vi "test_generic.vi"() -> ()   [LabVIEW 2010, in "GenericClock.lvclass"]
uses:
  GenericClock.lvclass
  common/classes/GenericComponent/GenericComponent/GenericComponent.lvclass
panel:
  in  "duty cycle":dbl[unit]
  in  "duration high":dbl[unit]
  in  "offset":dbl[unit]
  in  "create button":bool
  out "error out":errorcluster
  in  "stop":bool
  in  "start":bool
  in  "number of repetitions":i64=1000000000
  in  "pulse frequency":dbl[unit]=80000.0
  # "Test GenericClock"
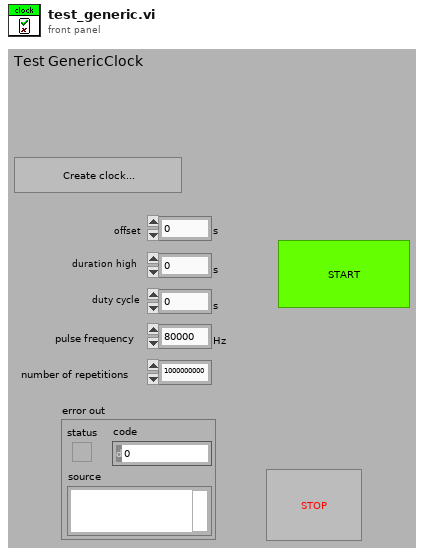
[diagram p1: front panel]
types:
  T1 = typedef "XComponentSpecification.xctl/data.ctl" = cluster{"class path":string, "configuration":string, "label":string, "settings name":string}
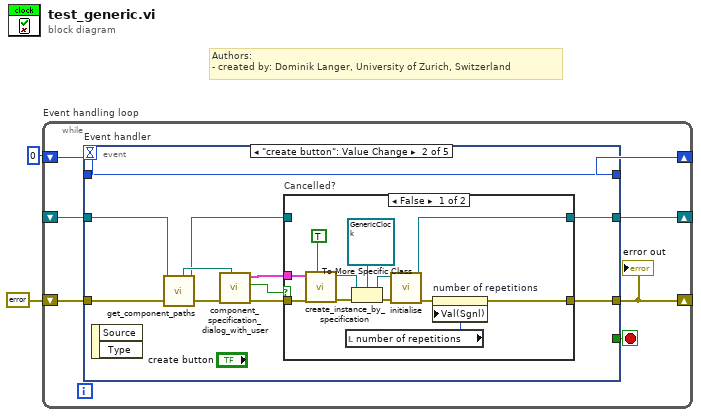
[diagram p0: block diagram]
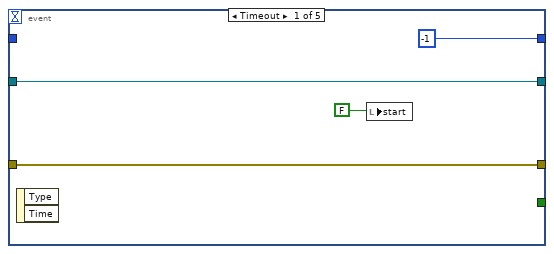
[diagram p2: hidden frame]
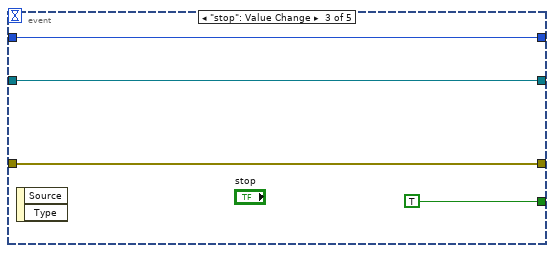
[diagram p4: hidden frame]
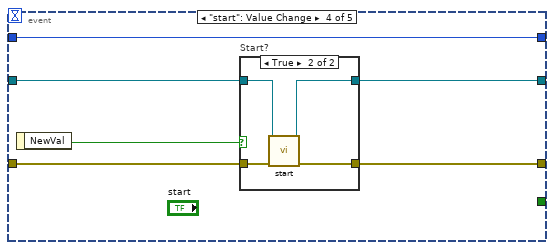
[diagram p5: hidden frame]
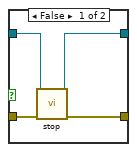
[diagram p6: hidden frame]
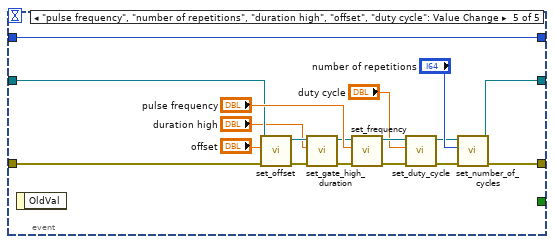
[diagram p7: hidden frame]
diagram:
  # "Authors: \n- created by: Dominik Langer, University of Zurich, Switzerland"
  n1 = while "Event handling loop" {
    shift-right: [w6] -> _
    shift-left: errorcluster {"status"=FALSE, "code"=0, "source"=""} ("error out") -> [w7]
    shift-right: [w5] -> _
    shift-left: _ -> [w9]
    shift-right: [w4] -> _
    shift-left: 0 -> [w8]
    stop <- w3 stop-if-true
    n2 = event "Event handler" shown="[1] \"create button\": Value Change" {
      selector: _ -> [_ _ _ _ _]
      dyn-events: _ -> [_ _ _ _ _]
      timeout: w8 -> [_ _ _ _ _]
      tunnel: w9 -> [w11 w18 w41 w46 w65]
      tunnel: w8 -> [_ w24 w40 w43 w70]
      tunnel: w7 -> [w10 w17 w42 w48 w68]
      tunnel: [w10 w23 w42 w45 w74] -> w6
      tunnel: [w11 w22 w41 w44 w73] -> w5
      tunnel: [-1 w24 w40 w43 w70] -> w4
      tunnel: [_ _ TRUE _ _] -> w3
      event Timeout {
        n3 = event-data() -> ()  [unwired: 3 out]
        n4 = local write "start"(FALSE) -> ()
      }
      event "create button": Value Change {
        n5 = event-data() -> ()  [unwired: 3 out]
        n6 = call-dynamic "get_component_paths.vi"("error in (no error)"=w17, "GenericComponent in"=w18) -> ("error out"=w16:errorcluster, "GenericComponent out"=w14:refnum<class "GenericClock.lvclass">, "component type directory"=w15:path)  [unwired: 4 in, 3 out]
        n7 = call "component_specification_dialog_with_user.vi"("start path"=w15, "error in (no error)"=w16) -> ("error out"=w21:errorcluster, "cancelled?"=w19:bool, "component specification out"=w20:T1)  [unwired: 7 in]
        n8 = case "Cancelled?" shown="False" w19 {
          tunnel: [w34 w37] -> w23
          tunnel: [w32 w38] -> w22
          tunnel: w21 -> [w26 w37]
          tunnel: w20 -> [w25 _]
          tunnel: w14 -> [_ w38]
          frame False {
            n9 = call "create_instance_by_specification.vi"("call constructor?"=TRUE, "error in (no error)"=w26, "component specification"=w25) -> ("error out"=w29:errorcluster, "GenericPlugin out"=w28:refnum<class "GenericComponent.lvclass">)  [unwired: 6 in, 1 out]
            n10 = local read "number of repetitions"() -> (w35:i64)
            n11 = To More Specific Class(target class=refnum<class "GenericClock.lvclass"> refnum ("GenericClock.lvclass"), reference=w28, error in=w29) -> (specific class reference=w30:refnum<class "GenericClock.lvclass">, error out=w31:errorcluster)
            n12 = call-dynamic "initialise.vi"("error in (no error)"=w31, "GenericPlugin in"=w30) -> ("error out"=w33:errorcluster, "GenericPlugin out"=w32:refnum<class "GenericClock.lvclass">)  [unwired: 8 out]
            n13 = property on="number of repetitions" class="DigNum (strict)"(error in=w33, "Val(Sgnl)"=w35) -> (error out=w34:errorcluster)  [unwired: 1 in, 1 out]
          }
          frame True {
          }
        }
      }
      event "stop": Value Change {
        n14 = event-data() -> ()  [unwired: 3 out]
      }
      event "start": Value Change {
        n15 = event-data() -> ("NewVal"=w47:bool)  [unwired: 1 out]
        n16 = case "Start?" shown="True" w47 {
          tunnel: w48 -> [w52 w56]
          tunnel: w46 -> [w51 w55]
          tunnel: [w49 w54] -> w45
          tunnel: [w50 w53] -> w44
          frame False {
            n17 = call-dynamic "stop.vi"("error in (no error)"=w52, "GenericClock in"=w51) -> ("error out"=w49:errorcluster, "GenericClock out"=w50:refnum<class "GenericClock.lvclass">)  [unwired: 8 out]
          }
          frame True {
            n18 = call-dynamic "start.vi"("error in (no error)"=w56, "GenericClock in"=w55) -> ("error out"=w54:errorcluster, "GenericClock out"=w53:refnum<class "GenericClock.lvclass">)  [unwired: 8 out]
          }
        }
      }
      event "pulse frequency", "number of repetitions", "duration high", "offset", "duty cycle": Value Change {
        n19 = event-data() -> ()  [unwired: 2 out]
        n20 = call-dynamic "set_offset.vi"("error in (no error)"=w68, "offset"="offset", "GenericClock.lvclass in"=w65) -> ("error out"=w67:errorcluster, "GenericClock.lvclass out"=w66:refnum<class "GenericClock.lvclass">)  [unwired: 7 out]
        n21 = call-dynamic "set_gate_high_duration.vi"("error in (no error)"=w67, "gate high duration"="duration high", "GenericClock.lvclass in"=w66) -> ("error out"=w69:errorcluster, "GenericClock.lvclass out"=w64:refnum<class "GenericClock.lvclass">)  [unwired: 7 out]
        n22 = call-dynamic "set_frequency.vi"("error in (no error)"=w69, "frequency"="pulse frequency", "GenericClock.lvclass in"=w64) -> ("error out"=w59:errorcluster, "GenericClock.lvclass out"=w61:refnum<class "GenericClock.lvclass">)  [unwired: 7 out]
        n23 = call-dynamic "set_duty_cycle.vi"("error in (no error)"=w59, "duty cycle"="duty cycle", "GenericClock.lvclass in"=w61) -> ("error out"=w58:errorcluster, "GenericClock.lvclass out"=w60:refnum<class "GenericClock.lvclass">)  [unwired: 7 out]
        n24 = call-dynamic "set_number_of_cycles.vi"("error in (no error)"=w58, "number of cycles"="number of repetitions", "GenericClock.lvclass in"=w60) -> ("error out"=w74:errorcluster, "GenericClock.lvclass out"=w73:refnum<class "GenericClock.lvclass">)  [unwired: 7 out]
      }
    }
    "error out" <- w6
  }
